vi "histung.vi"(6 "size":i32, 7 "cropresult":bool, 8 "step":dbl, 9 "start":dbl, 11 "X":dbl[](array[numeric])) -> (1 "X Values":dbl[](array[numeric]), 2 "H(x)":i32[](array[numeric]))   [LabVIEW 2012]
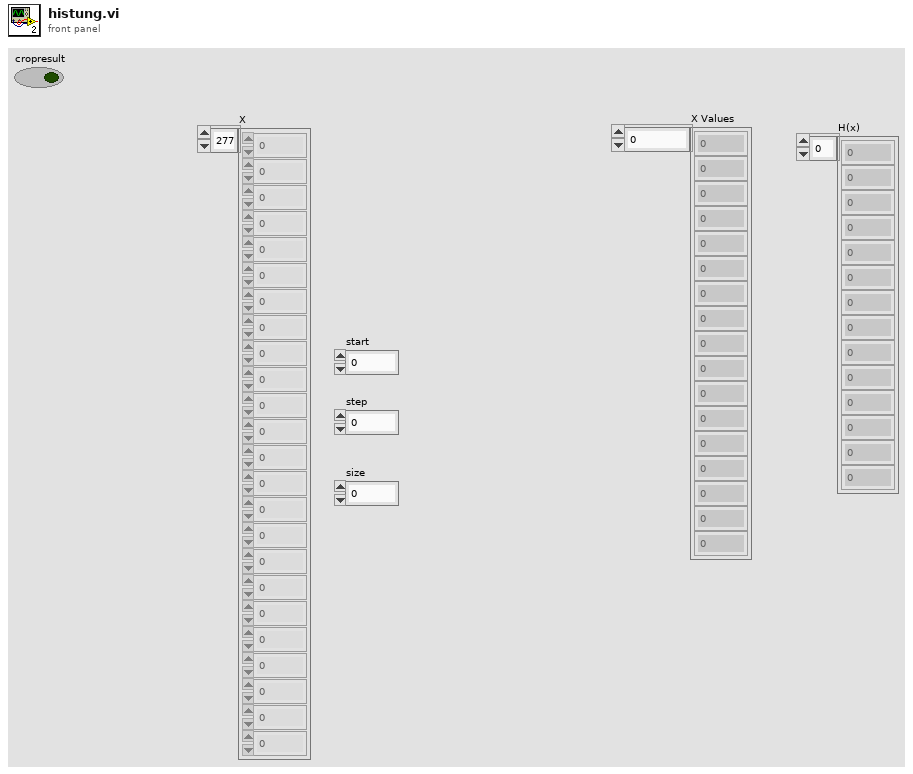
[diagram p1: front panel]
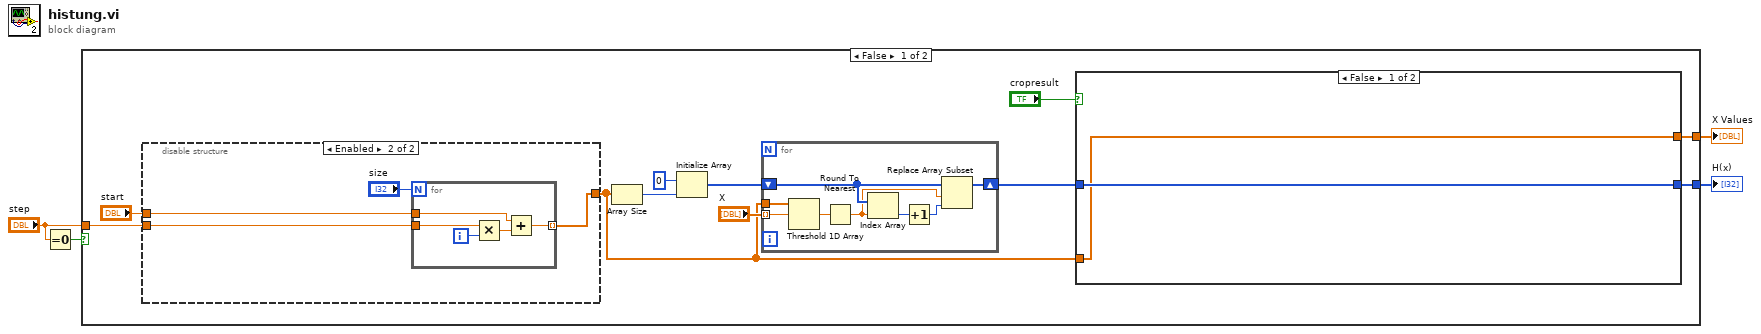
[diagram p0: block diagram]
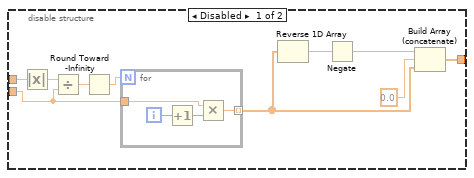
[diagram p2: hidden frame]
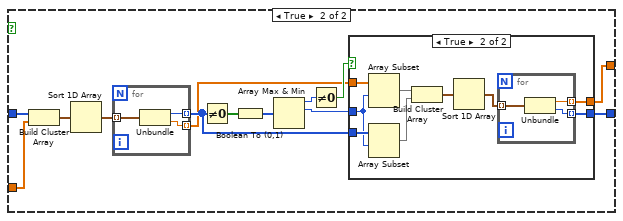
[diagram p3: hidden frame]
diagram:
  n1 = Equal To 0?(x="step") -> (x = 0?=w1:bool)
  n2 = case shown="False" w1 {
    tunnel: [w8 _] -> w4
    tunnel: [w7 _] -> w3
    tunnel: "step" -> [w6 _]
    frame False {
      n3 = disable-structure shown="Enabled" {
        disable-tunnel: "start" -> [w25 w32]
        disable-tunnel: [w19 w30] -> w9
        disable-tunnel: w6 -> [w16 w31]
        frame Disabled {
          n4 = Absolute Value(x=w25) -> (abs(x)=w18:dbl)
          n5 = Divide(x=w18, y=w16) -> (x/y=w24:dbl)
          n6 = Round Toward -Infinity(1:w24) -> (0:w17:dbl)
          n7 = for {
            N: w17 -> [_]
            tunnel: w16 -> [w27]
            tunnel: [w26] -> w20 mode=indexing
            i -> [w29]
            n8 = Increment(x=w29) -> (x+1=w28:i32)
            n9 = Multiply(x=w27, y=w28) -> (x*y=w26:dbl)
          }
          n10 = Reverse 1D Array(array=w20) -> (reversed array=w23:dbl[])
          n11 = Negate(x=w23) -> (-x=w22:dbl[])
          n12 = Build Array (concatenate)(w22, 0.0, w20) -> (w19:dbl[])
        }
        frame Enabled {
          n13 = for {
            N: "size" -> [_]
            tunnel: w32 -> [w35]
            tunnel: w31 -> [w37]
            tunnel: [w34] -> w30 mode=indexing
            i -> [w38]
            n14 = Multiply(x=w37, y=w38) -> (x*y=w36:dbl)
            n15 = Add(x=w35, y=w36) -> (x+y=w34:dbl)
          }
        }
      }
      n16 = Array Size(array=w9) -> (size(s)=w13:i32)
      n17 = Initialize Array(0, w13) -> (w11:i32[])
      n18 = for {
        tunnel: w9 -> [w76]
        tunnel: "X" -> [w75] mode=indexing
        shift-right: [w69] -> w10
        shift-left: w11 -> [w73]
        n19 = Threshold 1D Array(2:w75, 3:w76) -> (0:w74:dbl)  [unwired: 1 in]
        n20 = Round To Nearest(number=w74) -> (nearest integer value=w70:dbl)
        n21 = Index Array(array=w73, index=w70) -> (element=w72:i32)
        n22 = Increment(x=w72) -> (x+1=w71:i32)
        n23 = Replace Array Subset(array=w73, new element=w71, index=w70) -> (w69:i32[])
      }
      n24 = case shown="False" "cropresult" {
        tunnel: w10 -> [w40 w53]
        tunnel: w9 -> [w39 w52]
        tunnel: [w40 w42] -> w8
        tunnel: [w39 w41] -> w7
        frame False {
        }
        frame True {
          n25 = Build Cluster Array(w53, w52) -> (w51:cluster{i32, dbl}[])
          n26 = Sort 1D Array(array=w51) -> (sorted array=w50:cluster{i32, dbl}[])
          n27 = for {
            tunnel: w50 -> [w68] mode=indexing
            tunnel: [w67] -> w45 mode=indexing
            tunnel: [w66] -> w43 mode=indexing
            n28 = Unbundle(w68) -> (w67:i32, w66:dbl)
          }
          n29 = Not Equal To 0?(x=w45) -> (x != 0?=w49:bool[])
          n30 = Boolean To (0,1)(Boolean=w49) -> (0, 1=w48:i16[])
          n31 = Array Max & Min(array=w48) -> (max value=w47:i16, max index (indices)=w44:i32)  [unwired: 2 out]
          n32 = Not Equal To 0?(x=w47) -> (x != 0?=w46:bool)
          n33 = case shown="True" w46 {
            tunnel: w45 -> [_ w62]
            tunnel: w44 -> [_ w60]
            tunnel: w43 -> [_ w61]
            tunnel: [_ w55] -> w42
            tunnel: [_ w54] -> w41
            frame False {
            }
            frame True {
              n34 = Array Subset(array=w61, index=w60) -> (w58:dbl[])  [unwired: 1 in]
              n35 = Array Subset(array=w62, index=w60) -> (w57:i32[])  [unwired: 1 in]
              n36 = Build Cluster Array(w58, w57) -> (w59:cluster{dbl, i32}[])
              n37 = Sort 1D Array(array=w59) -> (sorted array=w56:cluster{dbl, i32}[])
              n38 = for {
                tunnel: w56 -> [w65] mode=indexing
                tunnel: [w64] -> w54 mode=indexing
                tunnel: [w63] -> w55 mode=indexing
                n39 = Unbundle(w65) -> (w64:dbl, w63:i32)
              }
            }
          }
        }
      }
    }
    frame True {
    }
  }
  "X Values" <- w3
  "H(x)" <- w4
